vi "PH_GUI.set color GUI object.vi"(0 "Visible? (true)":bool=TRUE, 1 "Disabled? (false)":bool, 2 "GUI object Ref":refnum<vi>, 3 "State":i32 caption="status", 4 "Blinking? (false)":bool, 5 "error in (no error)":errorcluster, 7 "Tip Strip (N/A)":string="N/A", 9 "Caption (N/A)":string="N/A") -> (19 "error out":errorcluster)   [LabVIEW 2014, in "PH_Common.lvlib"]
doc: "Sets value and more for the referenced GUI object."
uses:
  PH_Common.lvlib
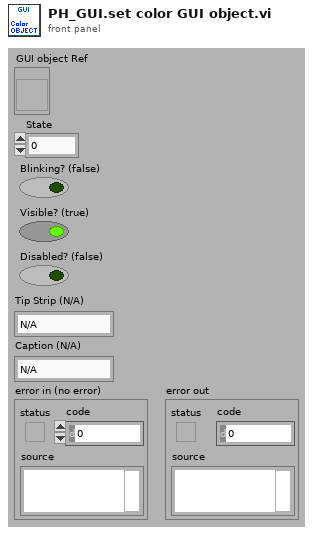
[diagram p1: front panel]
types:
  T1 = enum8{"Enabled", "Disabled", "Disabled and Grayed Out"}
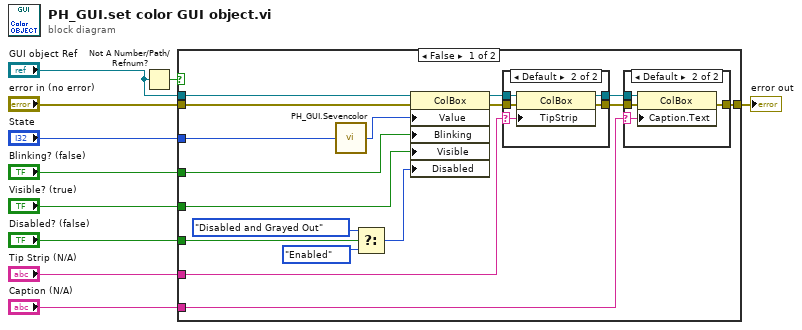
[diagram p0: block diagram]
diagram:
  n1 = Not A Number/Path/Refnum?(number/path/refnum="GUI object Ref") -> (NaN/Path/Refnum?=w6:bool)
  n2 = case shown="False" w6 {
    tunnel: "GUI object Ref" -> [w27 _]
    tunnel: "error in (no error)" -> [w26 w40]
    tunnel: [w16 w40] -> w9
    tunnel: "State" -> [w25 _]
    tunnel: "Blinking? (false)" -> [w23 _]
    tunnel: "Visible? (true)" -> [w22 _]
    tunnel: "Disabled? (false)" -> [w21 _]
    tunnel: "Tip Strip (N/A)" -> [w18 _]
    tunnel: "Caption (N/A)" -> [w14 _]
    frame False {
      n3 = call "PH_GUI.Sevencolor.vi"("State"=w25) -> ("Color Box"=w24:u32)
      n4 = Select(t=T1."Disabled and Grayed Out", s=w21, f=T1."Enabled" ("Disabled")) -> (s? t:f=w12:T1)
      n5 = property class="ColBox"(reference=w27, error in=w26, "Value"=w24, "Blinking"=w23, "Visible"=w22, "Disabled"=w12) -> (reference out=w19:refnum<vi>, error out=w20:errorcluster)
      n6 = case shown="Default" w18 {
        selector: w18 -> [_ w36]
        tunnel: w20 -> [w34 w39]
        tunnel: [w34 w38] -> w17
        tunnel: w19 -> [w33 w37]
        tunnel: [w33 w35] -> w15
        frame "", "N/A" {
        }
        frame Default {
          n7 = property class="ColBox"(reference=w37, error in=w39, "TipStrip"=w36) -> (reference out=w35:refnum<vi>, error out=w38:errorcluster)
        }
      }
      n8 = case shown="Default" w14 {
        selector: w14 -> [_ w29]
        tunnel: w17 -> [w28 w32]
        tunnel: [w28 w31] -> w16
        tunnel: w15 -> [_ w30]
        frame "", "N/A" {
        }
        frame Default {
          n9 = property class="ColBox"(reference=w30, error in=w32, "Caption.Text"=w29) -> (error out=w31:errorcluster)  [unwired: 1 out]
        }
      }
    }
    frame True {
    }
  }
  "error out" <- w9
